vi "close.vi"(8 "error in (no error)":errorcluster, 11 "HamegHMPSupply in":refnum<class "HamegHMPSupply.lvclass">) -> (0 "error out":errorcluster)   [LabVIEW 2009, in "Hardware.lvlib" / "Channels.lvlib" / "HamegHMPSupply.lvclass"]
doc: "Closes the analog output device."
uses:
  HamegHMPSupply.lvclass
  HamegHMPSupply.lvclass/HamegHMPSupply.ctl
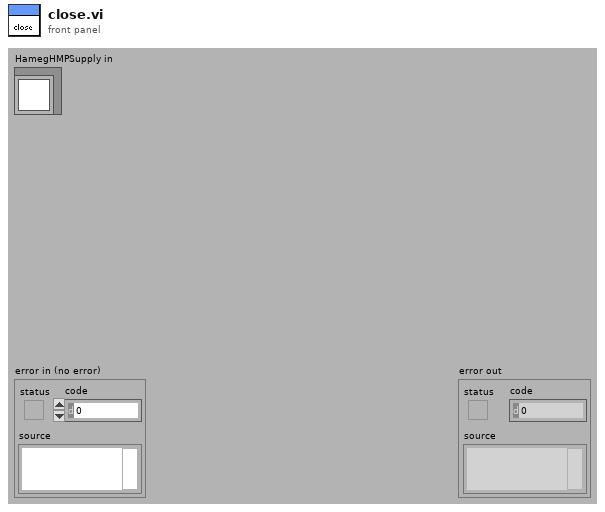
[diagram p1: front panel]
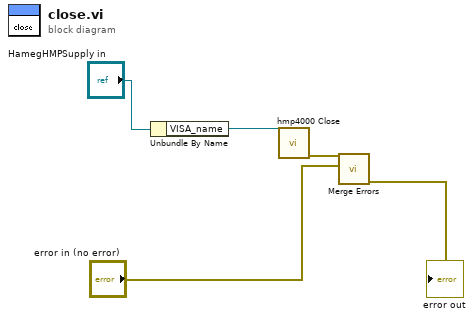
[diagram p0: block diagram]
diagram:
  n1 = Unbundle By Name("HamegHMPSupply in") -> ("VISA_name"=w4:refnum<visa-resource-name>)
  n2 = call <instrlib>:"hmp4000 Close.vi"("VISA resource name"=w4) -> ("error out"=w3:errorcluster)  [unwired: 10 in]
  n3 = call <vilib>:"Merge Errors.vi"("error in 2 (no error)"="error in (no error)", "error in 1 (no error)"=w3) -> ("error out"=→"error out":errorcluster)  [unwired: 5 in]
